vi "Interpret Status Word.vi"(8 "error in (no error)":errorcluster, 9 "Exit":bool, 10 "Status Word In":u16, 11 "State in":T1=enum."Shutdown - Normal") -> (0 "error out":errorcluster, 3 "State out":T1)   [LabVIEW 2016, in "Scan Engine Custom Device.lvlib" / "DS402.lvlib"]
uses:
  DS402.lvlib
  controls/state.ctl
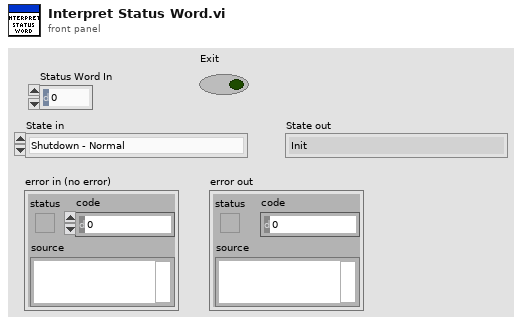
[diagram p1: front panel]
types:
  T1 = typedef "Scan Engine Custom Device.lvlib/DS402.lvlib/state.ctl" = enum16{"Init", "Not Ready to Switch On", "Read Status Word", "Switch on disabled", "Ready to switch on", "Switched on", "Operation enabled", "Fault", "Fault reaction active", "Quick stop active", "Shutdown - Bad State", "Shutdown - Error", "Shutdown - Normal", "Shutdown - Fault"}
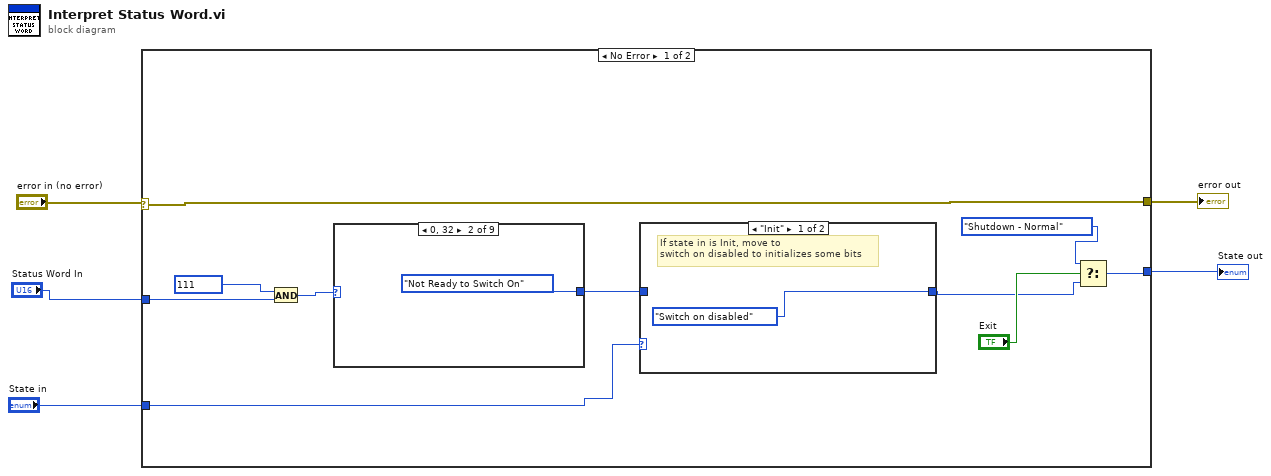
[diagram p0: block diagram]
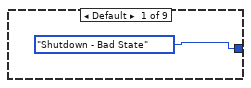
[diagram p3: hidden frame]
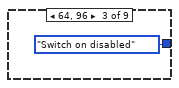
[diagram p4: hidden frame]
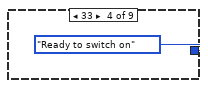
[diagram p5: hidden frame]
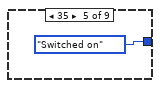
[diagram p6: hidden frame]
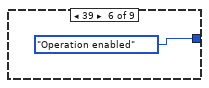
[diagram p7: hidden frame]
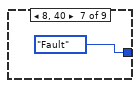
[diagram p8: hidden frame]
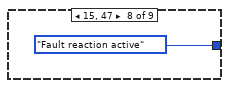
[diagram p9: hidden frame]
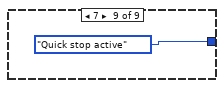
[diagram p10: hidden frame]
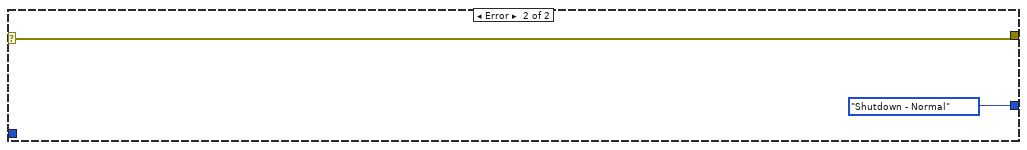
[diagram p11: hidden frame]
diagram:
  n1 = case shown="No Error" "error in (no error)" {
    selector: "error in (no error)" -> [w15 w28]
    tunnel: [w15 w28] -> w5
    tunnel: [w12 state."Shutdown - Normal" ("State out 2")] -> w1
    tunnel: "Status Word In" -> [w14 _]
    tunnel: "State in" -> [w9 _]
    frame No Error {
      n2 = And(x=u16 111, y=w14) -> (x .and. y?=w10:u16)
      n3 = case shown="0, 32" w10 {
        tunnel: [state."Shutdown - Bad State" ("State") state."Not Ready to Switch On" ("State") state."Switch on disabled" ("State") state."Ready to switch on" ("State") state."Switched on" ("State") state."Operation enabled" ("State") state."Fault" ("State") state."Fault reaction active" ("State") state."Quick stop active" ("State")] -> w8
        frame Default {
        }
        frame 0, 32 {
        }
        frame 64, 96 {
        }
        frame 33 {
        }
        frame 35 {
        }
        frame 39 {
        }
        frame 8, 40 {
        }
        frame 15, 47 {
        }
        frame 7 {
        }
      }
      n4 = case shown="\"Init\"" w9 {
        tunnel: [state."Switch on disabled" ("State") w17] -> w7
        tunnel: w8 -> [_ w17]
        frame "Init" {
          # "If state in is Init, move to \nswitch on disabled to initializes some bits"
        }
        frame Default {
        }
      }
      n5 = Select(t=state."Shutdown - Normal", s="Exit", f=w7) -> (s? t:f=w12:T1)
    }
    frame Error {
    }
  }
  "error out" <- w5
  "State out" <- w1
